vi "Model Create.vi"(8 "error in (no error)":errorcluster) -> (0 "error out":errorcluster)   [LabVIEW 2015]
uses:
  Control Button/Exit.ctl
  Control Button/Save.ctl
  Control Button/Delete.ctl
  <vilib>/addons/database/Connection.llb/DB Tools Open Connec (String).vi
  Galobal variable_TI.vi
  <vilib>/addons/database/_DB Variant To Data/Database Variant To Data.xnode
  <vilib>/addons/database/NI_Database_API.lvlib
panel:
  out "error out 2":errorcluster
  out "new path":path
  out "Program seq. Name":string[](array[string])
  out "error out":errorcluster
  in  "Program Name":string
  in  "Edit Name":string
  in  "Program List":i32(listbox)
  in  "Delete":T1
  in  "Save":T2
  in  "Exit":T3
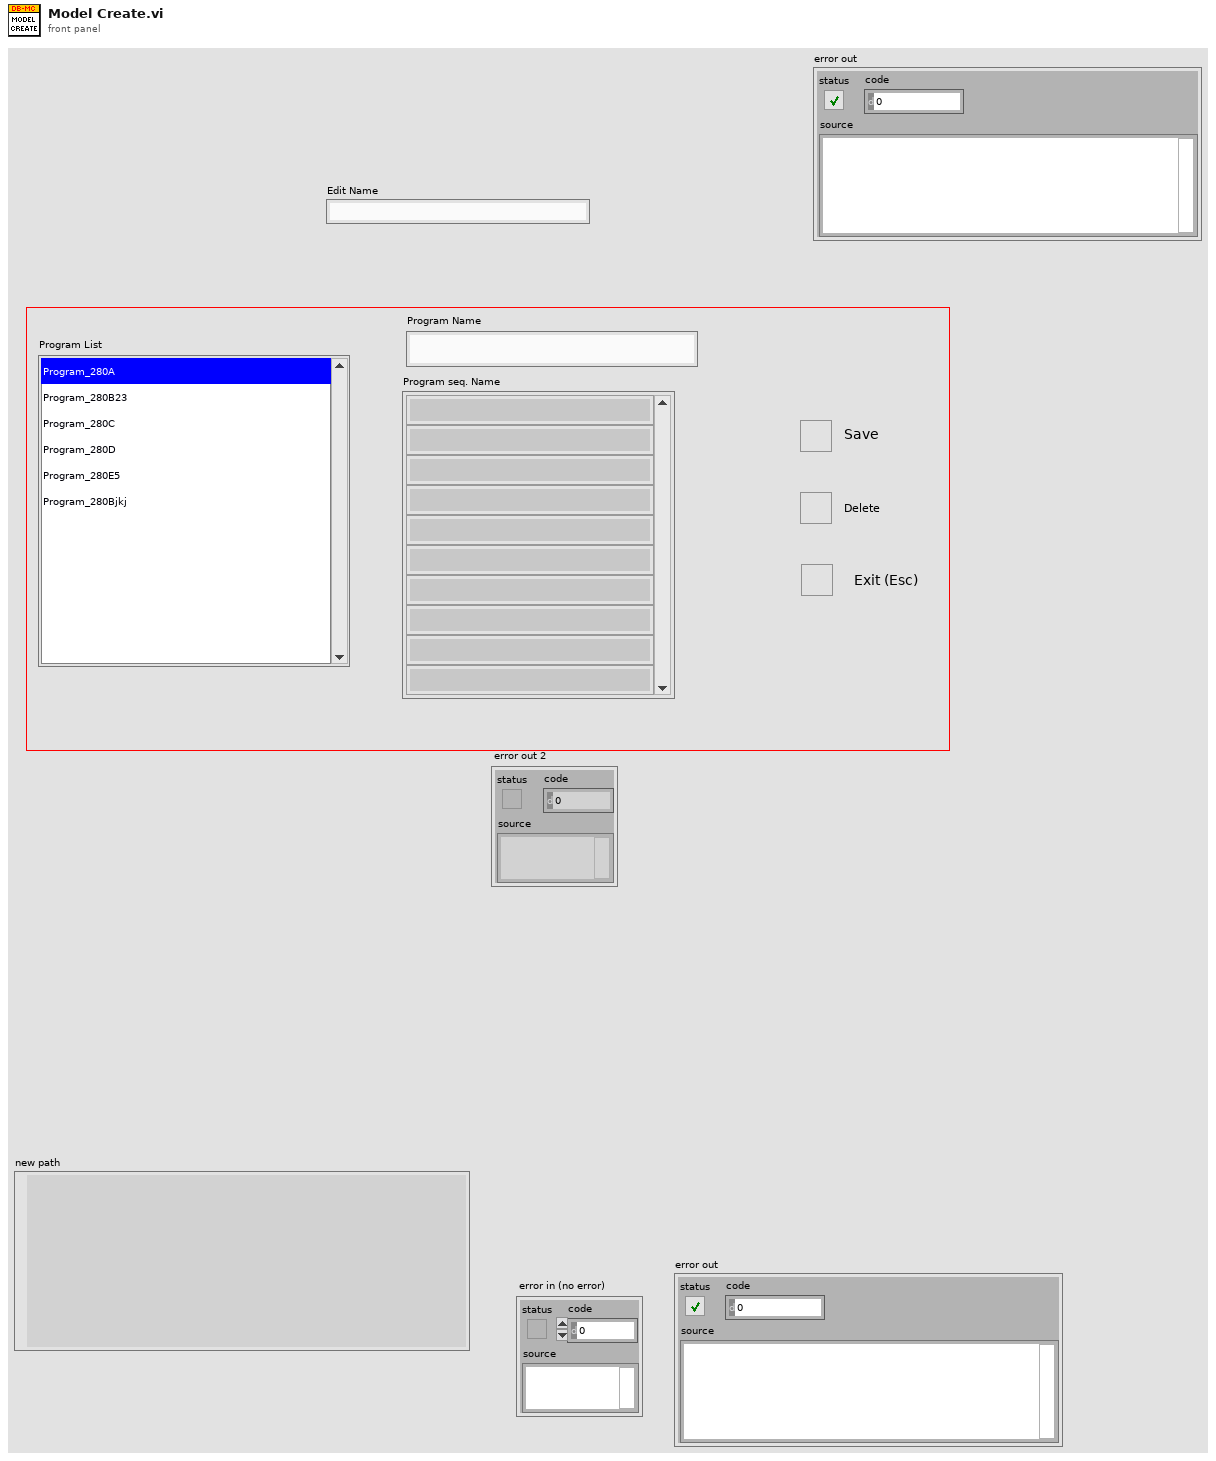
[diagram p1: front panel]
types:
  T1 = typedef "Delete.ctl" = bool
  T2 = typedef "Save.ctl" = bool
  T3 = typedef "Exit.ctl" = bool
  T4 = typedef "NI_Database_API.lvlib/Conn ObjectReference.ctl" = refnum<k1>
  T5 = enum16{"Left Button", "Center Button", "Right Button", "Window Close"}
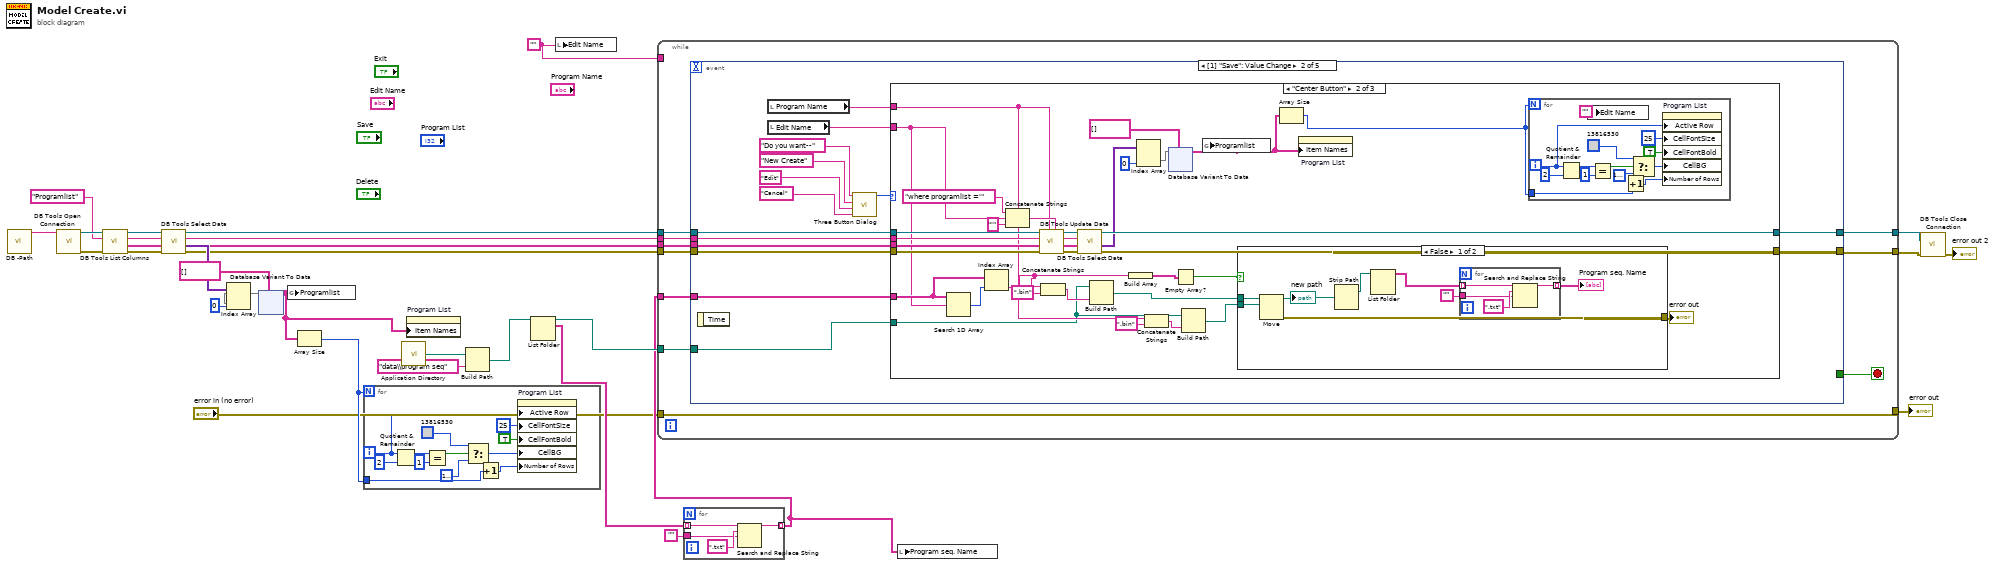
[diagram p0: block diagram]
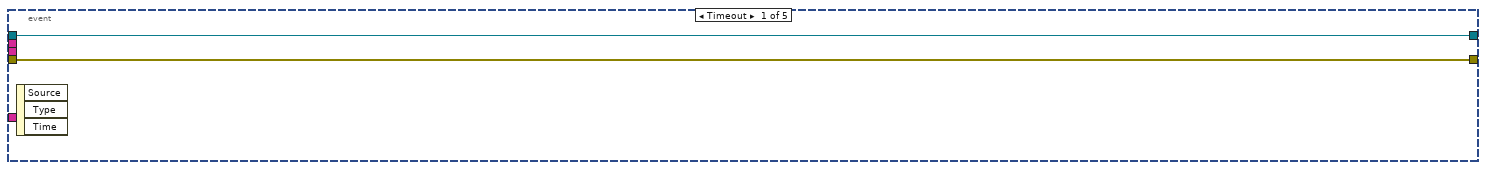
[diagram p2: hidden frame]
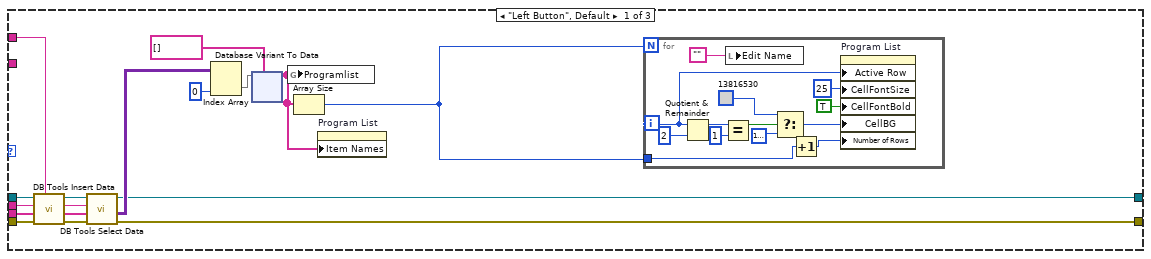
[diagram p3: hidden frame]
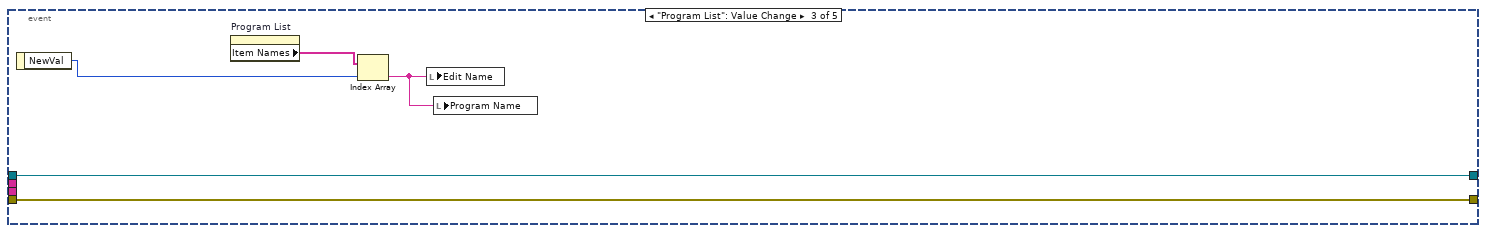
[diagram p6: hidden frame]
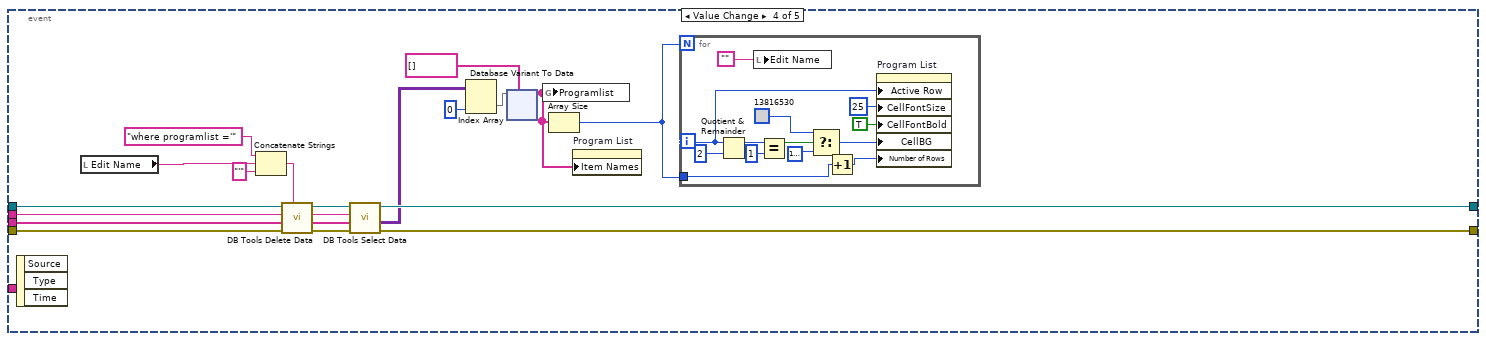
[diagram p7: hidden frame]
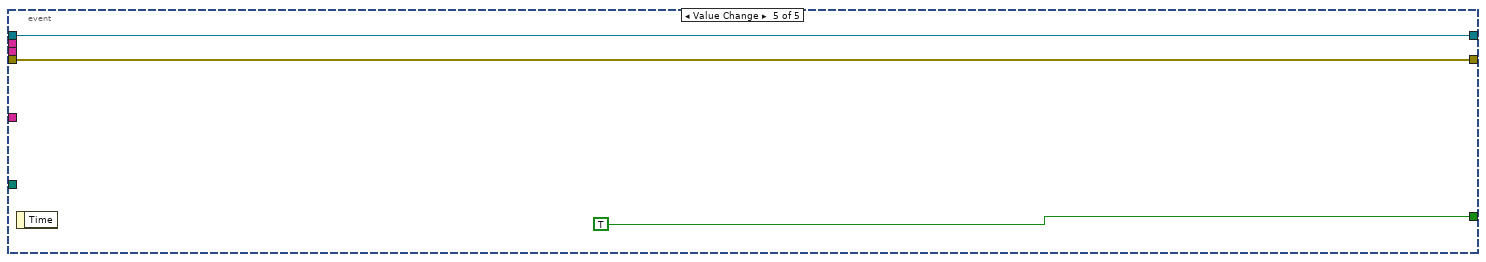
[diagram p8: hidden frame]
diagram:
  w11 = ""
  w14 = "Programlist" ("table")
  n1 = call "DB -Path.vi"() -> ("String"=w26:string)  [unwired: 11 in]
  n2 = call-poly <vilib>:"DB Tools Open Connection.vi"("connection information"=w26) -> ("error out"=w21:errorcluster, "connection reference"=w22:T4)  [unwired: 7 in]
  n3 = call <vilib>:"DB Tools List Columns.vi"("error in (no error)"=w21, "table"=w14, "connection reference"=w22) -> ("error out"=w19:errorcluster, "columns"=w15:string[], "connection reference out"=w20:T4)  [unwired: 1 in, 1 out]
  n4 = call <vilib>:"DB Tools Select Data.vi"("error in (no error)"=w19, "columns"=w15, "table"=w14, "connection reference"=w20) -> ("error out"=w16:errorcluster, "data"=w18:variant[][], "connection reference out"=w17:T4)  [unwired: 2 in]
  n5 = Index Array(array=w18, index (col)=0 ("disabled index (col)")) -> (element=w23:variant[])  [unwired: 1 in]
  n6 = xnode "Database Variant To Data"("database variant"=w23, "type"=string[] []) -> ("data"=w12:string[])  [unwired: 1 in, 1 out]
  n7 = global write "Galobal variable_TI.vi" "Programlist"(w12) -> ()
  n8 = Array Size(array=w12) -> (size(s)=w13:i32)
  n9 = for {
    N: w13 -> [_]
    tunnel: w13 -> [w30]
    i -> [w31]
    n10 = Quotient & Remainder(x=w31, y=2) -> (x-y*floor(x/y)=w39:i32)  [unwired: 1 out]
    n11 = Equal?(x=w39, y=1) -> (x = y?=w37:bool)
    n12 = Select(t=u32 13816530 ("Color Box"), s=w37, f=u32 16777225 ("Color Box")) -> (s? t:f=w34:u32)
    n13 = Increment(x=w30) -> (x+1=w29:i32)
    n14 = property on="Program List" class="LstBox (strict)"("Active Row"=w31, "CellFontSize"=u32 25 ("Active Row:Cell Font:Size"), "CellFontBold"=TRUE ("Active Row:Cell Font:Bold"), "CellBG"=w34, "Number of Rows"=w29) -> ()  [unwired: 2 in, 2 out]
  }
  n15 = call <vilib>:"Application Directory.vi"() -> ("Application Directory"=w28:path)
  n16 = property on="Program List" class="LstBox (strict)"("Item Names"=w12) -> ()  [unwired: 2 in, 2 out]
  n17 = Build Path(base path=w28, name or relative path="data\\program seq") -> (appended path=w10:path)
  n18 = List Folder(path=w10) -> (path out=w9:path, filenames=w8:string[])  [unwired: 3 in, 2 out]
  n19 = local write "Edit Name"(w11) -> ()
  n20 = for {
    tunnel: w8 -> [w44] mode=indexing
    tunnel: "" -> [w42]
    tunnel: [w41] -> w6 mode=indexing
    n21 = Search and Replace String(input string=w44, search string=".txt" ("replace string (\"\")"), replace string=w42) -> (result string=w41:string)  [unwired: 5 in, 3 out]
  }
  n22 = while {
    tunnel: w9 -> [w53]
    tunnel: w17 -> [w52]
    tunnel: w16 -> [w51]
    tunnel: w15 -> [w50]
    tunnel: w14 -> [w49]
    tunnel: [w48] -> w2
    tunnel: [w47] -> w3
    tunnel: w11 -> [_]
    tunnel: w6 -> [w46]
    tunnel: [w45] -> w5
    tunnel: "error in (no error)" -> [w45]
    stop <- w54 stop-if-true
    n23 = event shown="[1] \"Save\": Value Change" {
      selector: _ -> [_ _ _ _ _]
      dyn-events: _ -> [_ _ _ _ _]
      timeout: _ -> [_ _ _ _ _]
      tunnel: [_ _ _ _ TRUE] -> w54
      tunnel: w53 -> [_ w58 _ _ _]
      tunnel: w52 -> [w56 w66 w239 w257 w310]
      tunnel: w51 -> [w55 w65 w238 w256 w309]
      tunnel: w50 -> [_ w63 _ w252 _]
      tunnel: w49 -> [_ w64 _ w253 _]
      tunnel: [w56 w62 w239 w251 w310] -> w48
      tunnel: [w55 w61 w238 w250 w309] -> w47
      tunnel: w46 -> [_ w59 _ _ _]
      event Timeout {
        n24 = event-data() -> ()  [unwired: 1 in, 3 out]
      }
      event Value Change {
        n25 = event-data() -> ()  [unwired: 1 in, 1 out]
        n26 = local read "Program Name"() -> (w57:string)
        n27 = local read "Edit Name"() -> (w60:string)
        n28 = call <vilib>:"Three Button Dialog.vi"("Right Button Text (\"Cancel\")"="Cancel" ("Right Button Text (\"Cancel\")"), "Center Button Text (\"No\")"="Edit" ("Center Button Text (\"No\")"), "Left Button Text (\"Yes\")"="New Create" ("Left Button Text (\"Yes\")"), "message"="Do you want--" ("Left Button Text (\"Yes\")")) -> ("Which Button?"=w71:T5)  [unwired: 7 in]
        n29 = case shown="\"Center Button\"" w71 {
          tunnel: w66 -> [w86 w169 w234]
          tunnel: w65 -> [w85 w168 w233]
          tunnel: w64 -> [w82 w162 _]
          tunnel: w63 -> [w81 w161 _]
          tunnel: [w75 w160 w234] -> w62
          tunnel: [w74 w159 w233] -> w61
          tunnel: w60 -> [_ w148 _]
          tunnel: w59 -> [_ w152 _]
          tunnel: w58 -> [_ w141 _]
          tunnel: w57 -> [w72 w142 _]
          frame "Left Button", Default {
            n30 = call <vilib>:"DB Tools Insert Data.vi"("data"=w72, "error in (no error)"=w85, "columns"=w81, "table"=w82, "connection reference"=w86) -> ("error out"=w83:errorcluster, "connection reference out"=w84:T4)  [unwired: 5 in]
            n31 = call <vilib>:"DB Tools Select Data.vi"("error in (no error)"=w83, "columns"=w81, "table"=w82, "connection reference"=w84) -> ("error out"=w74:errorcluster, "data"=w77:variant[][], "connection reference out"=w75:T4)  [unwired: 2 in]
            n32 = Index Array(array=w77, index (col)=0 ("disabled index (col)")) -> (element=w80:variant[])  [unwired: 1 in]
            n33 = xnode "Database Variant To Data"("database variant"=w80, "type"=string[] []) -> ("data"=w73:string[])  [unwired: 1 in, 1 out]
            n34 = global write "Galobal variable_TI.vi" "Programlist"(w73) -> ()
            n35 = Array Size(array=w73) -> (size(s)=w76:i32)
            n36 = property on="Program List" class="LstBox (strict)"("Item Names"=w73) -> ()  [unwired: 2 in, 2 out]
            n37 = for {
              N: w76 -> [_]
              tunnel: w76 -> [w89]
              i -> [w90]
              n38 = Quotient & Remainder(x=w90, y=2) -> (x-y*floor(x/y)=w98:i32)  [unwired: 1 out]
              n39 = Equal?(x=w98, y=1) -> (x = y?=w96:bool)
              n40 = local write "Edit Name"("") -> ()
              n41 = Select(t=u32 13816530 ("Color Box"), s=w96, f=u32 16777225 ("Color Box")) -> (s? t:f=w93:u32)
              n42 = Increment(x=w89) -> (x+1=w88:i32)
              n43 = property on="Program List" class="LstBox (strict)"("Active Row"=w90, "CellFontSize"=u32 25 ("Active Row:Cell Font:Size"), "CellFontBold"=TRUE ("Active Row:Cell Font:Bold"), "CellBG"=w93, "Number of Rows"=w88) -> ()  [unwired: 2 in, 2 out]
            }
          }
          frame "Center Button" {
            n44 = Search 1D Array(1D array=w152, element=w148) -> (index of element=w151:i32)  [unwired: 1 in]
            n45 = Index Array(array=w152, index=w151) -> (element=w147:string)
            n46 = Concatenate Strings("where programlist ='" ("condition"), w148, "'" ("string")) -> (w167:string)
            n47 = call <vilib>:"DB Tools Update Data.vi"("condition"=w167, "data"=w142, "error in (no error)"=w168, "columns"=w161, "table"=w162, "connection reference"=w169) -> ("error out"=w163:errorcluster, "connection reference out"=w164:T4)  [unwired: 4 in]
            n48 = Concatenate Strings(w147, ".bin" ("string")) -> (w145:string)
            n49 = call <vilib>:"DB Tools Select Data.vi"("error in (no error)"=w163, "columns"=w161, "table"=w162, "connection reference"=w164) -> ("error out"=w159:errorcluster, "data"=w153:variant[][], "connection reference out"=w160:T4)  [unwired: 2 in]
            n50 = Build Path(base path=w141, name or relative path=w145) -> (appended path=w144:path)
            n51 = Build Array(w147) -> (w150:string[])
            n52 = Index Array(array=w153, index (col)=0 ("disabled index (col)")) -> (element=w158:variant[])  [unwired: 1 in]
            n53 = Concatenate Strings(w142, ".bin" ("string")) -> (w140:string)
            n54 = xnode "Database Variant To Data"("database variant"=w158, "type"=string[] []) -> ("data"=w154:string[])  [unwired: 1 in, 1 out]
            n55 = Empty Array?(array=w150) -> (empty?=w149:bool)
            n56 = Build Path(base path=w141, name or relative path=w140) -> (appended path=w139:path)
            n57 = global write "Galobal variable_TI.vi" "Programlist"(w154) -> ()
            n58 = case shown="False" w149 {
              tunnel: w144 -> [w177 _]
              tunnel: w139 -> [w176 _]
              tunnel: [w175 _] -> w138
              frame False {
                n59 = Move(source path=w177, 10:w176) -> (error out=w175:errorcluster, 3:w174:path)  [unwired: 3 in, 1 out]
                "new path" <- w174
                n60 = Strip Path(path=w174) -> (stripped path=w173:path)  [unwired: 1 out]
                n61 = List Folder(path=w173) -> (filenames=w171:string[])  [unwired: 3 in, 3 out]
                n62 = for {
                  tunnel: w171 -> [w181] mode=indexing
                  tunnel: "" -> [w179]
                  tunnel: [w178] -> w170 mode=indexing
                  n63 = Search and Replace String(input string=w181, search string=".txt" ("replace string (\"\")"), replace string=w179) -> (result string=w178:string)  [unwired: 5 in, 3 out]
                }
                "Program seq. Name" <- w170
              }
              frame True {
              }
            }
            "error out" <- w138
            n64 = Array Size(array=w154) -> (size(s)=w155:i32)
            n65 = property on="Program List" class="LstBox (strict)"("Item Names"=w154) -> ()  [unwired: 2 in, 2 out]
            n66 = for {
              N: w155 -> [_]
              tunnel: w155 -> [w184]
              i -> [w185]
              n67 = Quotient & Remainder(x=w185, y=2) -> (x-y*floor(x/y)=w193:i32)  [unwired: 1 out]
              n68 = local write "Edit Name"("") -> ()
              n69 = Equal?(x=w193, y=1) -> (x = y?=w191:bool)
              n70 = Increment(x=w184) -> (x+1=w183:i32)
              n71 = Select(t=u32 13816530 ("Color Box"), s=w191, f=u32 16777225 ("Color Box")) -> (s? t:f=w188:u32)
              n72 = property on="Program List" class="LstBox (strict)"("Active Row"=w185, "CellFontSize"=u32 25 ("Active Row:Cell Font:Size"), "CellFontBold"=TRUE ("Active Row:Cell Font:Bold"), "CellBG"=w188, "Number of Rows"=w183) -> ()  [unwired: 2 in, 2 out]
            }
          }
          frame "Right Button" {
          }
        }
      }
      event "Program List": Value Change {
        n73 = event-data() -> ("NewVal"=w236:i32)  [unwired: 1 in]
        n74 = property on="Program List" class="LstBox (strict)"() -> ("Item Names"=w237:string[])  [unwired: 2 in, 2 out]
        n75 = Index Array(array=w237, index=w236) -> (element=w235:string)
        n76 = local write "Edit Name"(w235) -> ()
        n77 = local write "Program Name"(w235) -> ()
      }
      event Value Change {
        n78 = event-data() -> ()  [unwired: 1 in, 3 out]
        n79 = local read "Edit Name"() -> (w240:string)
        n80 = Concatenate Strings("where programlist ='" ("condition"), w240, "'" ("string")) -> (w241:string)
        n81 = call <vilib>:"DB Tools Delete Data.vi"("condition"=w241, "error in (no error)"=w256, "table"=w253, "connection reference"=w257) -> ("error out"=w254:errorcluster, "connection reference out"=w255:T4)  [unwired: 6 in]
        n82 = call <vilib>:"DB Tools Select Data.vi"("error in (no error)"=w254, "columns"=w252, "table"=w253, "connection reference"=w255) -> ("error out"=w250:errorcluster, "data"=w244:variant[][], "connection reference out"=w251:T4)  [unwired: 2 in]
        n83 = Index Array(array=w244, index (col)=0 ("disabled index (col)")) -> (element=w249:variant[])  [unwired: 1 in]
        n84 = xnode "Database Variant To Data"("database variant"=w249, "type"=string[] []) -> ("data"=w245:string[])  [unwired: 1 in, 1 out]
        n85 = global write "Galobal variable_TI.vi" "Programlist"(w245) -> ()
        n86 = Array Size(array=w245) -> (size(s)=w246:i32)
        n87 = property on="Program List" class="LstBox (strict)"("Item Names"=w245) -> ()  [unwired: 2 in, 2 out]
        n88 = for {
          N: w246 -> [_]
          tunnel: w246 -> [w260]
          i -> [w261]
          n89 = Quotient & Remainder(x=w261, y=2) -> (x-y*floor(x/y)=w269:i32)  [unwired: 1 out]
          n90 = local write "Edit Name"("") -> ()
          n91 = Equal?(x=w269, y=1) -> (x = y?=w267:bool)
          n92 = Select(t=u32 13816530 ("Color Box"), s=w267, f=u32 16777225 ("Color Box")) -> (s? t:f=w264:u32)
          n93 = Increment(x=w260) -> (x+1=w259:i32)
          n94 = property on="Program List" class="LstBox (strict)"("Active Row"=w261, "CellFontSize"=u32 25 ("Active Row:Cell Font:Size"), "CellFontBold"=TRUE ("Active Row:Cell Font:Bold"), "CellBG"=w264, "Number of Rows"=w259) -> ()  [unwired: 2 in, 2 out]
        }
      }
      event Value Change {
        n95 = event-data() -> ()  [unwired: 1 in, 1 out]
      }
    }
  }
  "error out" <- w5
  n96 = local write "Program seq. Name"(w6) -> ()
  n97 = call <vilib>:"DB Tools Close Connection.vi"("error in (no error)"=w3, "connection reference"=w2) -> ("error out"=→"error out 2":errorcluster)  [unwired: 5 in]
